vi "HSDIO_6541_Main_StandAlone.vi"() -> ()   [LabVIEW 2015]
doc: "I Description: FOR TESTS PURPOSE ONLY\nThis VI inits a waveform generation session for HSDIO 6541. This is a basic example that shows how to setup the board in order to generate waveforms according to a script. \n\nII Instructions for Running:\n1. Start the VI and select any previously created sequence script.\n2. If software trigger is choosen, just click on the Send Software Trigger button to generate the sequence.\nIf not, connect an external TTL trigger to the PFI0 input pin of the HSDIO, and generation will start immediately after the next trigger pulse.\n\nIII Block Diagram Steps:\n1. Initialize for a generation session.\n2. Assign the specified channels in Channel List for dynamic operation.\n3. Configure the Sample clock to use the onboard clock, and configure the clock rate.\n\n\n\n1. Initialize for a generation session.\n2. Assign specified channels in Channel List for dynamic operation : all = \"\" (default)\n3. Sets the Idle State for when the generation has completed : NO !!\n4. Configure the Sample clock to use the onboard clock, and configure the clock rate.\n5. Set generation mode to Scripted.\n6. Configure the Script Trigger : change to Digital Edge if waiting for an external\n trigger, and link Rising Edge and source trigger commands.\n Use PFI0 with SMB wired to the board, or any PFIxx if connected to accessory.\n6. Initiate dynamic pattern generation.\n7. Wait until the generation is done.\n8. Close the generation session."
uses:
  controls/TEST_HSDIO_6541_Inputs.ctl
  controls/TEST_SEQUENCE_Inputs.ctl
  controls/SOFTWARE_Inputs.ctl
  <instrlib>/niHSDIO/niHSDIO.llb/niHSDIO_ctl Trigger SW - TrigIdentifier Values (Ring).ctl
  <instrlib>/niHSDIO/niHSDIO.llb/niHSDIO_ctl Trigger SW - TrigName Values (Ring).ctl
panel:
  in  "SOFTWARE Inputs":T1={"Application Directory"=path "D:/S.O.F.T.S/LABVIEW/PIL", "Resources Path"=path "D:/S.O.F.T.S/LABVIEW/PIL/resources", "Data Path"=path "D:/PIRENEA/DATA", "XML Path"=path "D:/PIRENEA/DATA", "XML File Filter"="*.xml", "Excit Scripts Path"=path "D:/PIRENEA/EXCIT_SCRIPTS", "Excit Scripts File Filter"="*.txt", "Excit Waveforms Path"=path "D:/PIRENEA/EXCIT_WFMS", "Excit Waveforms File Filter"="*.bin", "Sequence Scripts Path"=path "D:/PIRENEA/SEQUENCE_SCRIPTS", "Sequence Scripts File Filter"="*.txt", "Sequence Waveforms Path"=path "D:/PIRENEA/SEQUENCE_WFMS", "Sequence Waveforms File Filter"="*.bin", "Trapping Waveforms Path"=path "D:/PIRENEA/TRAPPING_WFMS", "Trapping Waveforms File Filter"="*.bin"} caption="SEQUENCE Inputs"
  out "Script text":string
  in  "SEQUENCE Inputs":T2={"Number Of Acquisitions "=0.0, "Number Of Accumulations"=0.0, "Number Of Loops"=0.0, "Scripts Path"=path "D:/PIRENEA/SEQUENCE_SCRIPTS", "Scripts File Filter"="*.txt", "Waveforms Path"=path "D:/PIRENEA/SEQUENCE_WFMS", "Waveforms File Filter"="*.bin"}
  in  "Use Software trigger":bool=TRUE
  in  "error in (no error)":errorcluster
  in  "HSDIO 6541 Inputs":T3={"Resource Name"=enum."SequencerHSDIO", "Clock Rate"=1000000.0, "Trigger Source"="PFI0"} {"Clock Rate" format="%.2p"}
  in  "Send Software Trigger":bool
  out "Ready for Trigger":bool
  in  "STOP ALL":bool
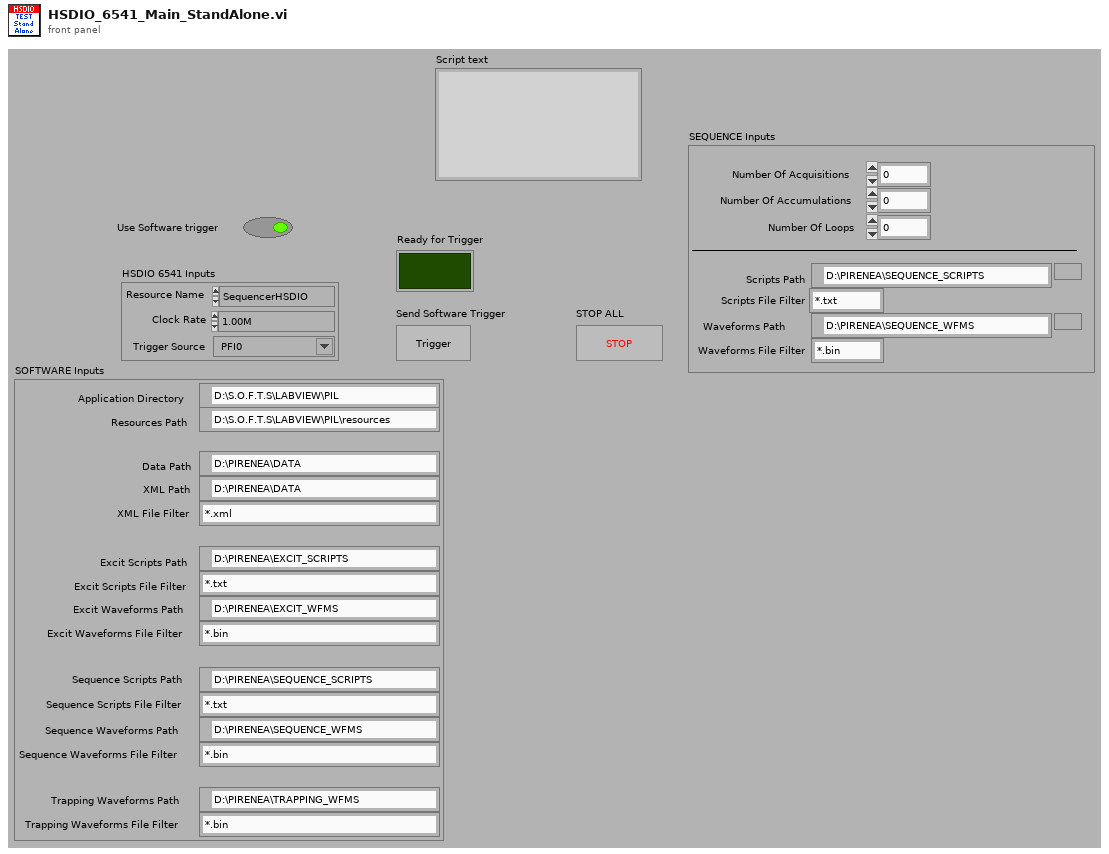
[diagram p1: front panel]
types:
  T1 = typedef "SOFTWARE_Inputs.ctl" = cluster{"Application Directory":path, "Resources Path":path, "Data Path":path, "XML Path":path, "XML File Filter":string, "Excit Scripts Path":path, "Excit Scripts File Filter":string, "Excit Waveforms Path":path, "Excit Waveforms File Filter":string, "Sequence Scripts Path":path, "Sequence Scripts File Filter":string, "Sequence Waveforms Path":path, "Sequence Waveforms File Filter":string, "Trapping Waveforms Path":path, "Trapping Waveforms File Filter":string}
  T2 = typedef "TEST_SEQUENCE_Inputs.ctl" = cluster{"Number Of Acquisitions ":dbl, "Number Of Accumulations":dbl, "Number Of Loops":dbl, "Scripts Path":path, "Scripts File Filter":string, "Waveforms Path":path, "Waveforms File Filter":string}
  T3 = typedef "TEST_HSDIO_6541_Inputs.ctl" = cluster{"Resource Name":enum16{"SequencerHSDIO", "SequencerHSDIO2"}, "Clock Rate":dbl, "Trigger Source":string}
  T4 = typedef "TEST_SEQUENCE_Outputs.ctl" = cluster{"Table of Waveforms":string[], "List of Waveforms":string, "Table of Scripts":string[], "List of Scripts":string, "Script Index":u32, "Script text":string, "FIFO used":i64, "FIFO max size":i32}
  T5 = typedef "niHSDIO_ctl Trigger SW - TrigIdentifier Values (Ring).ctl" = string
  T6 = typedef "niHSDIO_ctl Trigger SW - TrigName Values (Ring).ctl" = i32
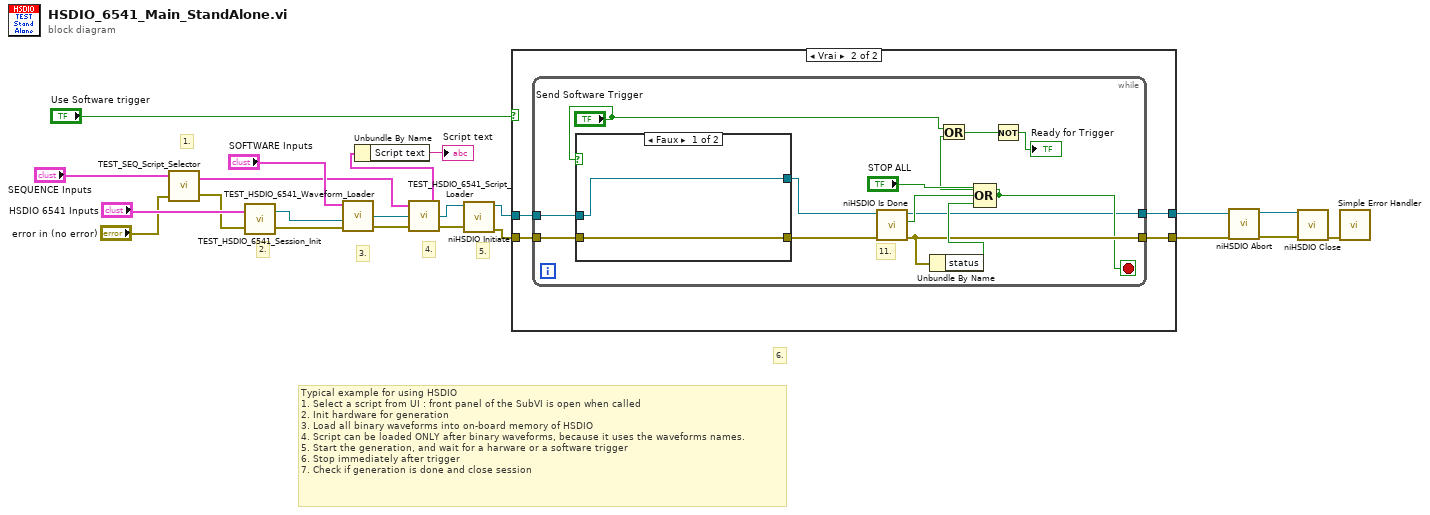
[diagram p0: block diagram]
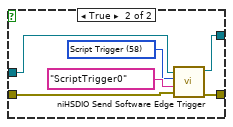
[diagram p3: hidden frame]
diagram:
  # "Typical example for using HSDIO\n1. Select a script from UI : front panel of the SubVI is open when called\n2. Init hardware for generation\n3. Load all binary waveforms into on-board memory of HSDIO\n4. Script can be loaded ONLY after binary waveforms, because it uses the waveforms names.\n5. Start the generation, and wait for a harware or a software trigger\n6. Stop immediately after trigger\n7. Check if generation is done and close session"
  # "6."
  # "5."
  # "4."
  # "3."
  # "2."
  # "1."
  n1 = call "TEST_SEQ_Script_Selector.vi"("error in (no error)"="error in (no error)", "SEQUENCE Inputs"="SEQUENCE Inputs") -> ("error out"=w12:errorcluster, "SEQUENCE Outputs"=w1:T4)  [unwired: 1 in]
  n2 = call "TEST_HSDIO_6541_Session_Init.vi"("error in (no error)"=w12, "HSDIO 6541 Inputs"="HSDIO 6541 Inputs") -> ("error out"=w11:errorcluster, "instrument handle out"=w18:refnum<k15>)
  n3 = call "TEST_HSDIO_6541_Waveform_Loader.vi"("error  in"=w11, "instrument handle in"=w18, "SOFTWARE Inputs"="SOFTWARE Inputs") -> ("error out"=w20:errorcluster, "instrument handle out"=w21:refnum<k15>)  [unwired: 2 in]
  n4 = call "TEST_HSDIO_6541_Script_Loader.vi"("error in (no error)"=w20, "instrument handle in"=w21, "SEQUENCE Outputs"=w1) -> ("error out"=w16:errorcluster, "instrument handle out"=w17:refnum<k15>, "SEQUENCE Outputs"=w9:T4)
  n5 = Unbundle By Name(w9) -> ("Script text"=→"Script text":string)
  n6 = call <instrlib>:"niHSDIO Initiate.vi"("error in (no error)"=w16, "instrument handle"=w17) -> ("error out"=w14:errorcluster, "instrument handle out"=w15:refnum<k15>)  [unwired: 8 in]
  n7 = case shown="Vrai" "Use Software trigger" {
    tunnel: [w23 w25] -> w7
    tunnel: [w24 w26] -> w5
    tunnel: w14 -> [w24 w28]
    tunnel: w15 -> [w23 w27]
    frame False {
    }
    frame True {
      n8 = while {
        tunnel: w28 -> [w40]
        tunnel: w27 -> [w39]
        tunnel: [w32] -> w26
        tunnel: [w29] -> w25
        stop <- w30 stop-if-true
        # "11."
        n9 = case shown="Faux" "Send Software Trigger" {
          tunnel: [w42 w49] -> w37
          tunnel: [w43 w48] -> w36
          tunnel: w40 -> [w43 w45]
          tunnel: w39 -> [w42 w44]
          frame False {
          }
          frame True {
            w46 = T6 58 items=["Start Trigger"=53, "Reference Trigger"=54, "Advance Trigger"=61, "Script Trigger"=58, "Stop Trigger"=82] ("trigger (start trigger)")
            n10 = call <instrlib>:"niHSDIO Send Software Edge Trigger.vi"("error in (no error)"=w45, "trigger identifier (none)"=T5 "ScriptTrigger0", "trigger (start trigger)"=w46, "instrument handle"=w44) -> ("error out"=w48:errorcluster, "instrument handle out"=w49:refnum<k15>)  [unwired: 6 in]
          }
        }
        n11 = call <instrlib>:"niHSDIO Is Done.vi"("error in (no error)"=w36, "instrument handle"=w37) -> ("error out"=w32:errorcluster, "done"=w34:bool, "instrument handle out"=w29:refnum<k15>)  [unwired: 7 in]
        n12 = Unbundle By Name(w32) -> ("status"=w33:bool)
        n13 = Compound Arithmetic op=OR ("Opérateur arithmétique")("STOP ALL", w34, w33) -> (w30:bool)
        n14 = Or(x="Send Software Trigger", y=w30) -> (x .or. y?=w38:bool)
        n15 = Not(x=w38) -> (.not. x?=→"Ready for Trigger":bool)
      }
    }
  }
  n16 = call <instrlib>:"niHSDIO Abort.vi"("error in (no error)"=w5, "instrument handle"=w7) -> ("error out"=w4:errorcluster, "instrument handle out"=w6:refnum<k15>)  [unwired: 8 in]
  n17 = call <instrlib>:"niHSDIO Close.vi"("error in (no error)"=w4, "instrument handle"=w6) -> ("error out"=w22:errorcluster)  [unwired: 9 in]
  n18 = call <vilib>:"Simple Error Handler.vi"("error in (no error)"=w22) -> ()  [unwired: 4 in, 5 out]
